vi "Aplicatie RN.vi"() -> ()   [LabVIEW 2024]
uses:
  <vilib>/picture/picture.llb/imagedata.ctl
panel:
  out "String":string
  in  "picture":picture
  out "new picture":picture
  out "image data":T1
  in  "Path":path
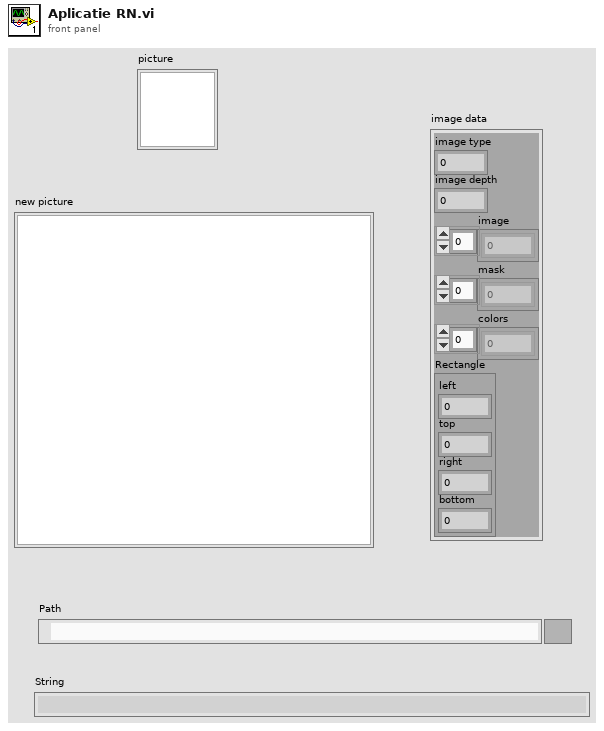
[diagram p1: front panel]
types:
  T1 = typedef "imagedata.ctl" = cluster{"image type":i32, "image depth":i32, "image":u8[], "mask":u8[], "colors":u32[], "Rectangle":cluster{"left":i16, "top":i16, "right":i16, "bottom":i16}}
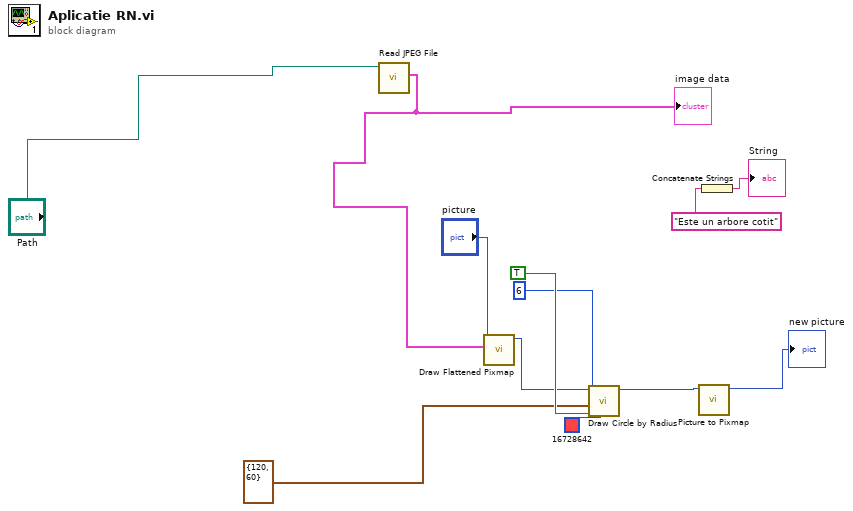
[diagram p0: block diagram]
diagram:
  n1 = call <vilib>:"Read JPEG File.vi"("path to JPEG file"="Path") -> ("image data"=w11:T1)  [unwired: 8 in, 2 out]
  "image data" <- w11
  n2 = call <vilib>:"Draw Flattened Pixmap.vi"("image data"=w11, "picture"="picture") -> ("new picture"=w8:picture)  [unwired: 7 in]
  n3 = call <vilib>:"Draw Circle by Radius.vi"("color(black)"=u32 16728642, "fill?(F)"=TRUE, "pixel center"=cluster{"horizontal":i16, "vertical":i16} {"horizontal"=120, "vertical"=60}, "radius"=i16 6, "picture"=w8) -> ("new picture"=w5:picture)  [unwired: 6 in]
  n4 = call <vilib>:"Picture to Pixmap.vi"("picture"=w5) -> ("new picture"=→"new picture":picture)  [unwired: 9 in, 1 out]
  n5 = Concatenate Strings("Este un arbore cotit") -> (→"String":string)
